vi "Get Thread ID Pool.vi"(11 "Transceiver Thread in":refnum<class "Transceiver Thread.lvclass">) -> (2 "Thread ID Pool":refnum<class "Pool ID.lvclass">, 3 "Transceiver Thread out":refnum<class "Transceiver Thread.lvclass">)   [LabVIEW 2017, in "Data Sharing Framework Engine.lvlib" / "Transceiver Thread.lvclass"]
uses:
  Transceiver Thread.lvclass
  Execution/Pool/Pool ID/Pool ID.lvclass
  Transceiver Thread.lvclass/Transceiver Thread.ctl
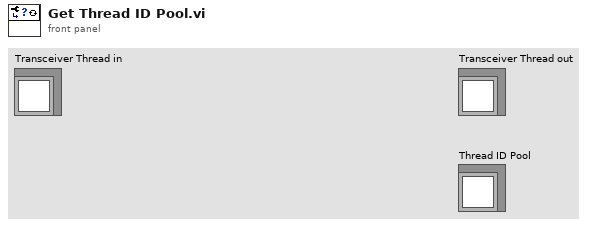
[diagram p1: front panel]
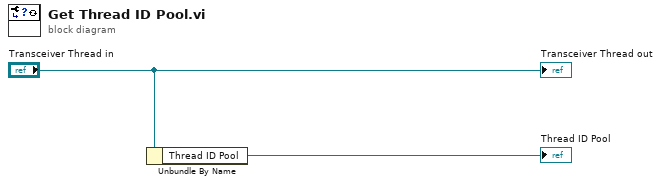
[diagram p0: block diagram]
diagram:
  n1 = Unbundle By Name("Transceiver Thread in") -> ("Thread ID Pool"=→"Thread ID Pool":refnum<class "Pool ID.lvclass">)
  "Transceiver Thread out" <- "Transceiver Thread in"
